vi "ZDataVIS_Update_Cursor_SingleArrayTest.vi"(7 "Field/Temperature 2":refnum<vi>, 8 "error in (no error)":errorcluster, 9 "Cursor Graph":refnum<vi>, 10 "Field / temp":i32, 11 "State Wire IN 2":T1={"Core"={"Current VI Reference"=refnum, "Close Panel on Exit?"=FALSE}, "Sweep Data Cluster"={"Vfast"=[[0.0, 0.25, 0.5, 0.75, 1.0, 1.25, 1.5, 1.75, 2.0, 2.25, 2.5, 2.75, 3.0, 3.25, 3.5, 3.75, 4.0, 4.25, 4.5, 4.75, 5.0, 5.25, 5.5, 5.75, 6.0, 6.25, 6.5, 6.75, 7.0, 7.25, 7.5, 7.75, 8.0, 8.25, 8.5, 8.75, 9.0, 9.25, 9.5, 9.75, 10.0, 10.25, 10.5, 10.75, 11.0, 11.25, 11.5, 11.75, 12.0, 12.25, 12.5, 12.75, 13.0, 13.25, 13.5, 13.75, 14.0, 14.25, 14.5, 14.75, 15.0], [0.0, 0.25, 0.5, 0.75, 1.0, 1.25, 1.5, 1.75, 2.0, 2.25, 2.5, 2.75, 3.0, 3.25, 3.5, 3.75, 4.0, 4.25, 4.5, 4.75, 5.0, 5.25, 5.5, 5.75, 6.0, 6.25, 6.5, 6.75, 7.0, 7.25, 7.5, 7.75, 8.0, 8.25, 8.5, 8.75, 9.0, 9.25, 9.5, 9.75, 10.0, 10.25, 10.5, 10.75, 11.0, 11.25, 11.5, 11.75, 12.0, 12.25, 12.5, 12.75, 13.0, 13.25, 13.5, 13.75, 14.0, 14.25, 14.5, 14.75, 15.0], [0.0, 0.25, 0.5, 0.75, 1.0, 1.25, 1.5, 1.75, 2.0, 2.25, 2.5, 2.75, 3.0, 3.25, 3.5, 3.75, 4.0, 4.25, 4.5, 4.75, 5.0, 5.25, 5.5, 5.75, 6.0, 6.25, 6.5, 6.75, 7.0, 7.25, 7.5, 7.75, 8.0, 8.25, 8.5, 8.75, 9.0, 9.25, 9.5, 9.75, 10.0, 10.25, 10.5, 10.75, 11.0, 11.25, 11.5, 11.75, 12.0, 12.25, 12.5, 12.75, 13.0, 13.25, 13.5, 13.75, 14.0, 14.25, 14.5, 14.75, 15.0], [0.0, 0.25, 0.5, 0.75, 1.0, 1.25, 1.5, 1.75, 2.0, 2.25, 2.5, 2.75, 3.0, 3.25, 3.5, 3.75, 4.0, 4.25, 4.5, 4.75, 5.0, 5.25, 5.5, 5.75, 6.0, 6.25, 6.5, 6.75, 7.0, 7.25, 7.5, 7.75, 8.0, 8.25, 8.5, 8.75, 9.0, 9.25, 9.5, 9.75, 10.0, 10.25, 10.5, 10.75, 11.0, 11.25, 11.5, 11.75, 12.0, 12.25, 12.5, 12.75, 13.0, 13.25, 13.5, 13.75, 14.0, 14.25, 14.5, 14.75, 15.0], [0.0, 0.25, 0.5, 0.75, 1.0, 1.25, 1.5, 1.75, 2.0, 2.25, 2.5, 2.75, 3.0, 3.25, 3.5, 3.75, 4.0, 4.25, 4.5, 4.75, 5.0, 5.25, 5.5, 5.75, 6.0, 6.25, 6.5, 6.75, 7.0, 7.25, 7.5, 7.75, 8.0, 8.25, 8.5, 8.75, 9.0, 9.25, 9.5, 9.75, 10.0, 10.25, 10.5, 10.75, 11.0, 11.25, 11.5, 11.75, 12.0, 12.25, 12.5, 12.75, 13.0, 13.25, 13.5, 13.75, 14.0, 14.25, 14.5, 14.75, 15.0], [0.0, 0.25, 0.5, 0.75, 1.0, 1.25, 1.5, 1.75, 2.0, 2.25, 2.5, 2.75, 3.0, 3.25, 3.5, 3.75, 4.0, 4.25, 4.5, 4.75, 5.0, 5.25, 5.5, 5.75, 6.0, 6.25, 6.5, 6.75, 7.0, 7.25, 7.5, 7.75, 8.0, 8.25, 8.5, 8.75, 9.0, 9.25, 9.5, 9.75, 10.0, 10.25, 10.5, 10.75, 11.0, 11.25, 11.5, 11.75, 12.0, 12.25, 12.5, 12.75, 13.0, 13.25, 13.5, 13.75, 14.0, 14.25, 14.5, 14.75, 15.0], [0.0, 0.25, 0.5, 0.75, 1.0, 1.25, 1.5, 1.75, 2.0, 2.25, 2.5, 2.75, 3.0, 3.25, 3.5, 3.75, 4.0, 4.25, 4.5, 4.75, 5.0, 5.25, 5.5, 5.75, 6.0, 6.25, 6.5, 6.75, 7.0, 7.25, 7.5, 7.75, 8.0, 8.25, 8.5, 8.75, 9.0, 9.25, 9.5, 9.75, 10.0, 10.25, 10.5, 10.75, 11.0, 11.25, 11.5, 11.75, 12.0, 12.25, 12.5, 12.75, 13.0, 13.25, 13.5, 13.75, 14.0, 14.25, 14.5, 14.75, 15.0], [0.0, 0.25, 0.5, 0.75, 1.0, 1.25, 1.5, 1.75, 2.0, 2.25, 2.5, 2.75, 3.0, 3.25, 3.5, 3.75, 4.0, 4.25, 4.5, 4.75, 5.0, 5.25, 5.5, 5.75, 6.0, 6.25, 6.5, 6.75, 7.0, 7.25, 7.5, 7.75, 8.0, 8.25, 8.5, 8.75, 9.0, 9.25, 9.5, 9.75, 10.0, 10.25, 10.5, 10.75, 11.0, 11.25, 11.5, 11.75, 12.0, 12.25, 12.5, 12.75, 13.0, 13.25, 13.5, 13.75, 14.0, 14.25, 14.5, 14.75, 15.0]], "Vslow"=[0.0, 1.0, 2.0, 3.0, 4.0, 5.0, 6.0, 7.0], "Vslowest"=[7.00003046875], "Comments"="      #Vslow/#Vfast/# of IV curves/BT offset/#discarded IV curves/Manual offset:\n /8/61/1/0/0/0    \n#of fields: 1    \nField period 1 \nDecimate point 1.000000 \nScan names \nDAQ_Vbg\nB\nB \n IGOR\nX// Date: 7/19/2018 6:19 PM\nX// SA03008H\nX// \nX// Source 2 Drain 28 (lockin 1 and 7)\nX// Gohm resistor, sweep BG\nX// \nX// 50mV AC -150mV DC for the IV sweep\nX// \nX// 0 to 15 slowly at 0.25 V step sizes\nX// Stepping B 0-7 @ 1T steps\n\nX// B_Field=7.000000\n\nX// \n\nX// B_Field_Rate=0.400000\n\nX// \n\nX// DAQ_Vbg=15.000000\n\nX// \nX// B= 7.000030\n\n\n\n\n\n\n\n\n\n\n\n\n\n\n\n\n\n\n\n\n\n\n\n\n\n\n\n\n\n\n\n\n\n\n\n\n\n\n\n\nX \nX Display/R 'time.SA03008H.20180718.000487'\nX AppendToGraph 'temp.SA03008H.20180718.000487'\nX AppendToGraph 'B.SA03008H.20180718.000487'\nX AppendToGraph 'Vsource.SA03008H.20180718.000487'\nX AppendToGraph 'Lockin0.SA03008H.20180718.000487'\nX AppendToGraph 'Lockin1.SA03008H.20180718.000487'\nX AppendToGraph 'Lockin2.SA03008H.20180718.000487'\nX AppendToGraph 'Lockin3.SA03008H.20180718.000487'\nX AppendToGraph 'Lockin4.SA03008H.20180718.000487'\nX AppendToGraph 'Lockin5.SA03008H.20180718.000487'\nX AppendToGraph 'B_rate.SA03008H.20180718.000487'\nX AppendToGraph 'DC0.SA03008H.20180718.000487'\nX AppendToGraph 'DC1.SA03008H.20180718.000487'\nX AppendToGraph 'DC2.SA03008H.20180718.000487'\nX AppendToGraph 'DC3.SA03008H.20180718.000487'\nX AppendToGraph 'DC4.SA03008H.20180718.000487'\nX AppendToGraph 'DC5.SA03008H.20180718.000487'\nX AppendToGraph 'DC6.SA03008H.20180718.000487'\nX AppendToGraph 'DC7.SA03008H.20180718.000487'\nX Label bottom \"x label\"\nX Label left \"y label\"\nX ModifyGraph rgb('time.SA03008H.20180718.000487')=(65280,0,0)\nX ModifyGraph rgb('temp.SA03008H.20180718.000487')=(65280,18432,0)\nX ModifyGraph rgb('B.SA03008H.20180718.000487')=(65280,36864,0)\nX ModifyGraph rgb('Vsource.SA03008H.20180718.000487')=(65280,55296,0)\nX ModifyGraph rgb('Lockin0.SA03008H.20180718.000487')=(57344,65280,0)\nX ModifyGraph rgb('Lockin1.SA03008H.20180718.000487')=(37376,65280,0)\nX ModifyGraph rgb('Lockin2.SA03008H.20180718.000487')=(18944,65280,0)\nX ModifyGraph rgb('Lockin3.SA03008H.20180718.000487')=(512,65280,0)\nX ModifyGraph rgb('Lockin4.SA03008H.20180718.000487')=(0,65280,17920)\nX ModifyGraph rgb('Lockin5.SA03008H.20180718.000487')=(0,65280,36352)\nX ModifyGraph rgb('B_rate.SA03008H.20180718.000487')=(0,65280,54784)\nX ModifyGraph rgb('DC0.SA03008H.20180718.000487')=(0,57856,65280)\nX ModifyGraph rgb('DC1.SA03008H.20180718.000487')=(0,39424,65280)\nX ModifyGraph rgb('DC2.SA03008H.20180718.000487')=(0,20992,65280)\nX ModifyGraph rgb('DC3.SA03008H.20180718.000487')=(0,2560,65280)\nX ModifyGraph rgb('DC4.SA03008H.20180718.000487')=(17408,0,65280)\nX ModifyGraph rgb('DC5.SA03008H.20180718.000487')=(35840,0,65280)\nX ModifyGraph rgb('DC6.SA03008H.20180718.000487')=(54272,0,65280)\nX ModifyGraph rgb('DC7.SA03008H.20180718.000487')=(65280,0,58368)\nX Legend/C/N=text0/J \"\\\\s('time.SA03008H.20180718.000487') time\\r\\\\s('temp.SA03008H.20180718.000487') temp\\r\\\\s('B.SA03008H.20180718.000487') B\\r\\\\s('Vsource.SA03008H.20180718.000487') Vsource\\r\\\\s('Lockin0.SA03008H.20180718.000487') Lockin0\\r\\\\s('Lockin1.SA03008H.20180718.000487') Lockin1\\r\\\\s('Lockin2.SA03008H.20180718.000487') Lockin2\\r\\\\s('Lockin3.SA03008H.20180718.000487') Lockin3\\r\\\\s('Lockin4.SA03008H.20180718.000487') Lockin4\\r\\\\s('Lockin5.SA03008H.20180718.000487') Lockin5\\r\\\\s('B_rate.SA03008H.20180718.000487') B_rate\\r\\\\s('DC0.SA03008H.20180718.000487') DC0\\r\\\\s('DC1.SA03008H.20180718.000487') DC1\\r\\\\s('DC2.SA03008H.20180718.000487') DC2\\r\\\\s('DC3.SA03008H.20180718.000487') DC3\\r\\\\s('DC4.SA03008H.20180718.000487') DC4\\r\\\\s('DC5.SA03008H.20180718.000487') DC5\\r\\\\s('DC6.SA03008H.20180718.000487') DC6\\r\\\\s('DC7.SA03008H.20180718.000487') DC7\"\nX ModifyGraph mirror(bottom)=1\nX ModifyGraph width=216\nX ModifyGraph height={Aspect,0.6}\nX ModifyGraph Log(bottom)=0\nX ModifyGraph Log(left)=0\nX \n", "Scan names"=["DAQ_Vbg", "B", "B"]}, "Cursor Info"={"Fast Index"=[33.0, 33.0, 33.0, 33.0, 33.0, 33.0, 33.0, 33.0], "Slow Index"=4.0, "Slow Indices"=[0.0, 1.0, 2.0, 3.0, 4.0, 5.0, 6.0, 7.0], "Raw Cursor Position"={"X"=8.146964856230031, "Y"=4.108108108108109}, "Field / temp"=0}, "Scan names"=["DAQ_Vbg", "B", "B"], "Data DVR"=refnum}) -> (0 "error out":errorcluster, 1 "Field":dbl=4.108108108108109, 2 "slowest":dbl=7.00003046875, 3 "State Wire IN 3":T1={"Core"={"Current VI Reference"=refnum, "Close Panel on Exit?"=FALSE}, "Sweep Data Cluster"={"Vfast"=[[0.0, 0.25, 0.5, 0.75, 1.0, 1.25, 1.5, 1.75, 2.0, 2.25, 2.5, 2.75, 3.0, 3.25, 3.5, 3.75, 4.0, 4.25, 4.5, 4.75, 5.0, 5.25, 5.5, 5.75, 6.0, 6.25, 6.5, 6.75, 7.0, 7.25, 7.5, 7.75, 8.0, 8.25, 8.5, 8.75, 9.0, 9.25, 9.5, 9.75, 10.0, 10.25, 10.5, 10.75, 11.0, 11.25, 11.5, 11.75, 12.0, 12.25, 12.5, 12.75, 13.0, 13.25, 13.5, 13.75, 14.0, 14.25, 14.5, 14.75, 15.0], [0.0, 0.25, 0.5, 0.75, 1.0, 1.25, 1.5, 1.75, 2.0, 2.25, 2.5, 2.75, 3.0, 3.25, 3.5, 3.75, 4.0, 4.25, 4.5, 4.75, 5.0, 5.25, 5.5, 5.75, 6.0, 6.25, 6.5, 6.75, 7.0, 7.25, 7.5, 7.75, 8.0, 8.25, 8.5, 8.75, 9.0, 9.25, 9.5, 9.75, 10.0, 10.25, 10.5, 10.75, 11.0, 11.25, 11.5, 11.75, 12.0, 12.25, 12.5, 12.75, 13.0, 13.25, 13.5, 13.75, 14.0, 14.25, 14.5, 14.75, 15.0], [0.0, 0.25, 0.5, 0.75, 1.0, 1.25, 1.5, 1.75, 2.0, 2.25, 2.5, 2.75, 3.0, 3.25, 3.5, 3.75, 4.0, 4.25, 4.5, 4.75, 5.0, 5.25, 5.5, 5.75, 6.0, 6.25, 6.5, 6.75, 7.0, 7.25, 7.5, 7.75, 8.0, 8.25, 8.5, 8.75, 9.0, 9.25, 9.5, 9.75, 10.0, 10.25, 10.5, 10.75, 11.0, 11.25, 11.5, 11.75, 12.0, 12.25, 12.5, 12.75, 13.0, 13.25, 13.5, 13.75, 14.0, 14.25, 14.5, 14.75, 15.0], [0.0, 0.25, 0.5, 0.75, 1.0, 1.25, 1.5, 1.75, 2.0, 2.25, 2.5, 2.75, 3.0, 3.25, 3.5, 3.75, 4.0, 4.25, 4.5, 4.75, 5.0, 5.25, 5.5, 5.75, 6.0, 6.25, 6.5, 6.75, 7.0, 7.25, 7.5, 7.75, 8.0, 8.25, 8.5, 8.75, 9.0, 9.25, 9.5, 9.75, 10.0, 10.25, 10.5, 10.75, 11.0, 11.25, 11.5, 11.75, 12.0, 12.25, 12.5, 12.75, 13.0, 13.25, 13.5, 13.75, 14.0, 14.25, 14.5, 14.75, 15.0], [0.0, 0.25, 0.5, 0.75, 1.0, 1.25, 1.5, 1.75, 2.0, 2.25, 2.5, 2.75, 3.0, 3.25, 3.5, 3.75, 4.0, 4.25, 4.5, 4.75, 5.0, 5.25, 5.5, 5.75, 6.0, 6.25, 6.5, 6.75, 7.0, 7.25, 7.5, 7.75, 8.0, 8.25, 8.5, 8.75, 9.0, 9.25, 9.5, 9.75, 10.0, 10.25, 10.5, 10.75, 11.0, 11.25, 11.5, 11.75, 12.0, 12.25, 12.5, 12.75, 13.0, 13.25, 13.5, 13.75, 14.0, 14.25, 14.5, 14.75, 15.0], [0.0, 0.25, 0.5, 0.75, 1.0, 1.25, 1.5, 1.75, 2.0, 2.25, 2.5, 2.75, 3.0, 3.25, 3.5, 3.75, 4.0, 4.25, 4.5, 4.75, 5.0, 5.25, 5.5, 5.75, 6.0, 6.25, 6.5, 6.75, 7.0, 7.25, 7.5, 7.75, 8.0, 8.25, 8.5, 8.75, 9.0, 9.25, 9.5, 9.75, 10.0, 10.25, 10.5, 10.75, 11.0, 11.25, 11.5, 11.75, 12.0, 12.25, 12.5, 12.75, 13.0, 13.25, 13.5, 13.75, 14.0, 14.25, 14.5, 14.75, 15.0], [0.0, 0.25, 0.5, 0.75, 1.0, 1.25, 1.5, 1.75, 2.0, 2.25, 2.5, 2.75, 3.0, 3.25, 3.5, 3.75, 4.0, 4.25, 4.5, 4.75, 5.0, 5.25, 5.5, 5.75, 6.0, 6.25, 6.5, 6.75, 7.0, 7.25, 7.5, 7.75, 8.0, 8.25, 8.5, 8.75, 9.0, 9.25, 9.5, 9.75, 10.0, 10.25, 10.5, 10.75, 11.0, 11.25, 11.5, 11.75, 12.0, 12.25, 12.5, 12.75, 13.0, 13.25, 13.5, 13.75, 14.0, 14.25, 14.5, 14.75, 15.0], [0.0, 0.25, 0.5, 0.75, 1.0, 1.25, 1.5, 1.75, 2.0, 2.25, 2.5, 2.75, 3.0, 3.25, 3.5, 3.75, 4.0, 4.25, 4.5, 4.75, 5.0, 5.25, 5.5, 5.75, 6.0, 6.25, 6.5, 6.75, 7.0, 7.25, 7.5, 7.75, 8.0, 8.25, 8.5, 8.75, 9.0, 9.25, 9.5, 9.75, 10.0, 10.25, 10.5, 10.75, 11.0, 11.25, 11.5, 11.75, 12.0, 12.25, 12.5, 12.75, 13.0, 13.25, 13.5, 13.75, 14.0, 14.25, 14.5, 14.75, 15.0]], "Vslow"=[0.0, 1.0, 2.0, 3.0, 4.0, 5.0, 6.0, 7.0], "Vslowest"=[7.00003046875], "Comments"="      #Vslow/#Vfast/# of IV curves/BT offset/#discarded IV curves/Manual offset:\n /8/61/1/0/0/0    \n#of fields: 1    \nField period 1 \nDecimate point 1.000000 \nScan names \nDAQ_Vbg\nB\nB \n IGOR\nX// Date: 7/19/2018 6:19 PM\nX// SA03008H\nX// \nX// Source 2 Drain 28 (lockin 1 and 7)\nX// Gohm resistor, sweep BG\nX// \nX// 50mV AC -150mV DC for the IV sweep\nX// \nX// 0 to 15 slowly at 0.25 V step sizes\nX// Stepping B 0-7 @ 1T steps\n\nX// B_Field=7.000000\n\nX// \n\nX// B_Field_Rate=0.400000\n\nX// \n\nX// DAQ_Vbg=15.000000\n\nX// \nX// B= 7.000030\n\n\n\n\n\n\n\n\n\n\n\n\n\n\n\n\n\n\n\n\n\n\n\n\n\n\n\n\n\n\n\n\n\n\n\n\n\n\n\n\nX \nX Display/R 'time.SA03008H.20180718.000487'\nX AppendToGraph 'temp.SA03008H.20180718.000487'\nX AppendToGraph 'B.SA03008H.20180718.000487'\nX AppendToGraph 'Vsource.SA03008H.20180718.000487'\nX AppendToGraph 'Lockin0.SA03008H.20180718.000487'\nX AppendToGraph 'Lockin1.SA03008H.20180718.000487'\nX AppendToGraph 'Lockin2.SA03008H.20180718.000487'\nX AppendToGraph 'Lockin3.SA03008H.20180718.000487'\nX AppendToGraph 'Lockin4.SA03008H.20180718.000487'\nX AppendToGraph 'Lockin5.SA03008H.20180718.000487'\nX AppendToGraph 'B_rate.SA03008H.20180718.000487'\nX AppendToGraph 'DC0.SA03008H.20180718.000487'\nX AppendToGraph 'DC1.SA03008H.20180718.000487'\nX AppendToGraph 'DC2.SA03008H.20180718.000487'\nX AppendToGraph 'DC3.SA03008H.20180718.000487'\nX AppendToGraph 'DC4.SA03008H.20180718.000487'\nX AppendToGraph 'DC5.SA03008H.20180718.000487'\nX AppendToGraph 'DC6.SA03008H.20180718.000487'\nX AppendToGraph 'DC7.SA03008H.20180718.000487'\nX Label bottom \"x label\"\nX Label left \"y label\"\nX ModifyGraph rgb('time.SA03008H.20180718.000487')=(65280,0,0)\nX ModifyGraph rgb('temp.SA03008H.20180718.000487')=(65280,18432,0)\nX ModifyGraph rgb('B.SA03008H.20180718.000487')=(65280,36864,0)\nX ModifyGraph rgb('Vsource.SA03008H.20180718.000487')=(65280,55296,0)\nX ModifyGraph rgb('Lockin0.SA03008H.20180718.000487')=(57344,65280,0)\nX ModifyGraph rgb('Lockin1.SA03008H.20180718.000487')=(37376,65280,0)\nX ModifyGraph rgb('Lockin2.SA03008H.20180718.000487')=(18944,65280,0)\nX ModifyGraph rgb('Lockin3.SA03008H.20180718.000487')=(512,65280,0)\nX ModifyGraph rgb('Lockin4.SA03008H.20180718.000487')=(0,65280,17920)\nX ModifyGraph rgb('Lockin5.SA03008H.20180718.000487')=(0,65280,36352)\nX ModifyGraph rgb('B_rate.SA03008H.20180718.000487')=(0,65280,54784)\nX ModifyGraph rgb('DC0.SA03008H.20180718.000487')=(0,57856,65280)\nX ModifyGraph rgb('DC1.SA03008H.20180718.000487')=(0,39424,65280)\nX ModifyGraph rgb('DC2.SA03008H.20180718.000487')=(0,20992,65280)\nX ModifyGraph rgb('DC3.SA03008H.20180718.000487')=(0,2560,65280)\nX ModifyGraph rgb('DC4.SA03008H.20180718.000487')=(17408,0,65280)\nX ModifyGraph rgb('DC5.SA03008H.20180718.000487')=(35840,0,65280)\nX ModifyGraph rgb('DC6.SA03008H.20180718.000487')=(54272,0,65280)\nX ModifyGraph rgb('DC7.SA03008H.20180718.000487')=(65280,0,58368)\nX Legend/C/N=text0/J \"\\\\s('time.SA03008H.20180718.000487') time\\r\\\\s('temp.SA03008H.20180718.000487') temp\\r\\\\s('B.SA03008H.20180718.000487') B\\r\\\\s('Vsource.SA03008H.20180718.000487') Vsource\\r\\\\s('Lockin0.SA03008H.20180718.000487') Lockin0\\r\\\\s('Lockin1.SA03008H.20180718.000487') Lockin1\\r\\\\s('Lockin2.SA03008H.20180718.000487') Lockin2\\r\\\\s('Lockin3.SA03008H.20180718.000487') Lockin3\\r\\\\s('Lockin4.SA03008H.20180718.000487') Lockin4\\r\\\\s('Lockin5.SA03008H.20180718.000487') Lockin5\\r\\\\s('B_rate.SA03008H.20180718.000487') B_rate\\r\\\\s('DC0.SA03008H.20180718.000487') DC0\\r\\\\s('DC1.SA03008H.20180718.000487') DC1\\r\\\\s('DC2.SA03008H.20180718.000487') DC2\\r\\\\s('DC3.SA03008H.20180718.000487') DC3\\r\\\\s('DC4.SA03008H.20180718.000487') DC4\\r\\\\s('DC5.SA03008H.20180718.000487') DC5\\r\\\\s('DC6.SA03008H.20180718.000487') DC6\\r\\\\s('DC7.SA03008H.20180718.000487') DC7\"\nX ModifyGraph mirror(bottom)=1\nX ModifyGraph width=216\nX ModifyGraph height={Aspect,0.6}\nX ModifyGraph Log(bottom)=0\nX ModifyGraph Log(left)=0\nX \n", "Scan names"=["DAQ_Vbg", "B", "B"]}, "Cursor Info"={"Fast Index"=[33.0, 33.0, 33.0, 33.0, 33.0, 33.0, 33.0, 33.0], "Slow Index"=4.0, "Slow Indices"=[0.0, 1.0, 2.0, 3.0, 4.0, 5.0, 6.0, 7.0], "Raw Cursor Position"={"X"=8.146964856230031, "Y"=4.108108108108109}, "Field / temp"=0}, "Scan names"=["DAQ_Vbg", "B", "B"], "Data DVR"=refnum})   [LabVIEW 2016]
uses:
  ZDataVIS_StateWire.ctl
  <vilib>/Utility/miscctls.llb/LVPointDoubleTypeDef.ctl
panel:
  # "cursor x"
  # "cursor y"
  # "cursor x"
  # "cursor y"
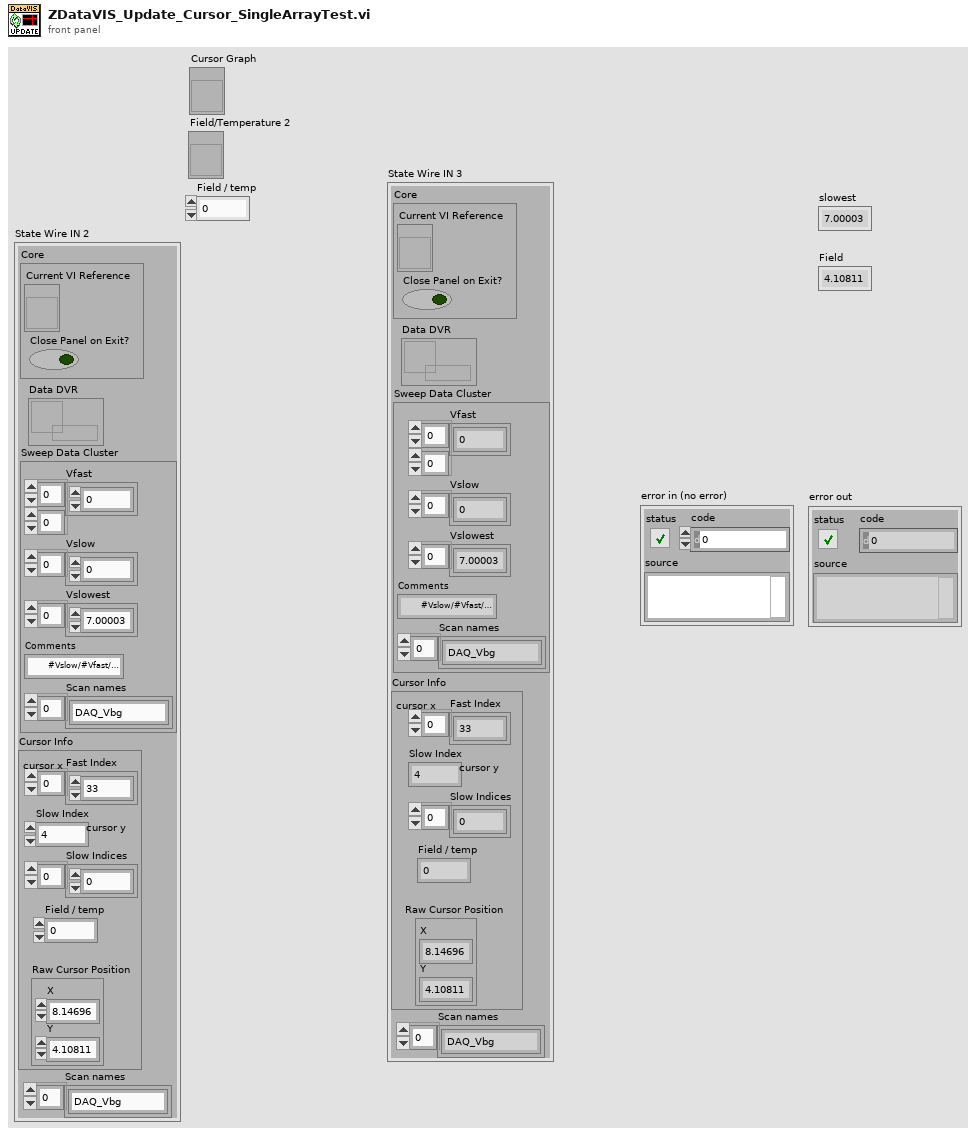
[diagram p1: front panel]
types:
  T1 = typedef "ZDataVIS_StateWire.ctl" = cluster{"Core":cluster{"Current VI Reference":refnum<vi>, "Close Panel on Exit?":bool}, "Sweep Data Cluster":cluster{"Vfast":dbl[][], "Vslow":dbl[], "Vslowest":dbl[], "Comments":string, "Scan names":string[]}, "Cursor Info":cluster{"Fast Index":dbl[], "Slow Index":dbl, "Slow Indices":dbl[], "Raw Cursor Position":T2, "Field / temp":i32}, "Scan names":string[], "Data DVR":refnum<data-value>}
  T2 = typedef "LVPointDoubleTypeDef.ctl" = cluster{"X":dbl, "Y":dbl}
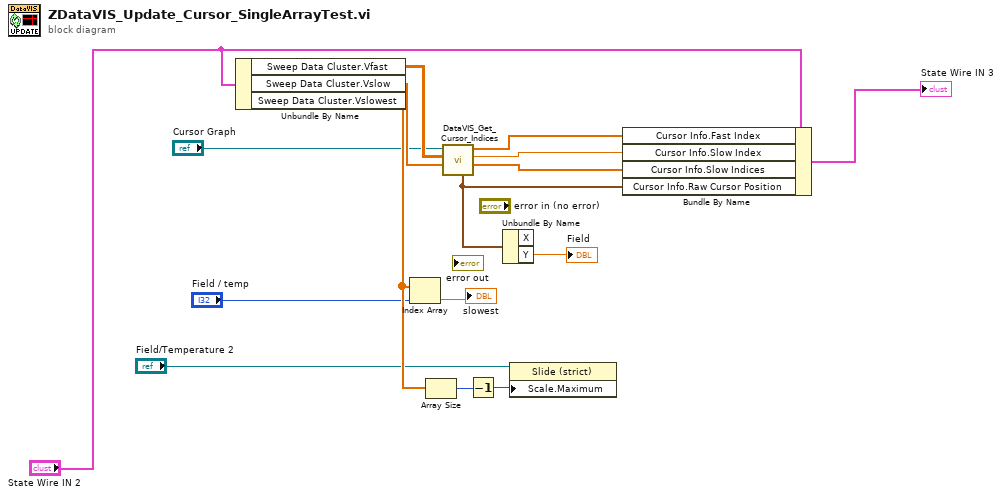
[diagram p0: block diagram]
diagram:
  n1 = Unbundle By Name("State Wire IN 2") -> ("Sweep Data Cluster.Vfast"=w16:dbl[][], "Sweep Data Cluster.Vslow"=w15:dbl[], "Sweep Data Cluster.Vslowest"=w10:dbl[])
  n2 = Index Array(array=w10, index="Field / temp") -> (element=→"slowest":dbl)
  n3 = Array Size(array=w10) -> (size(s)=w14:i32)
  n4 = call "DataVIS_Get_Cursor_Indices.vi"("Vslow"=w15, "Vfast"=w16, "Cursor Graph"="Cursor Graph") -> ("Slow Indices"=w7:dbl[], "Slow Index (Cursor Y)"=w8:dbl, "Fast Index (Cursor X) (IDK why it's an array)"=w9:dbl[], "Raw Cursor Position"=w6:T2)  [unwired: 4 in, 1 out]
  n5 = Decrement(x=w14) -> (x-1=w13:i32)
  n6 = Unbundle By Name(w6) -> ("Y"=→"Field":dbl)  [unwired: 1 out]
  n7 = property on="Property Node" class="Slide (strict)"(reference="Field/Temperature 2", "Scale.Maximum"=w13) -> ()  [unwired: 1 in, 2 out]
  n8 = Bundle By Name(cluster="State Wire IN 2", "Cursor Info.Fast Index"=w9, "Cursor Info.Slow Index"=w8, "Cursor Info.Slow Indices"=w7, "Cursor Info.Raw Cursor Position"=w6) -> (→"State Wire IN 3":T1)
